vi "UTILITY General Time Header.vi"(6 "precision (6)":i16=6, 7 "Add Elapsed Time (hrs)":bool, 8 "Error In":errorcluster, 9 "Software Elapsed Time":dbl format="%<%H:%M:%S>t", 10 "Elapsed Time":dbl, 11 "Add Software Elapsed Time":bool) -> (0 "Error Out":errorcluster, 3 "Total Array":string[][](array[string]))   [LabVIEW 2020]
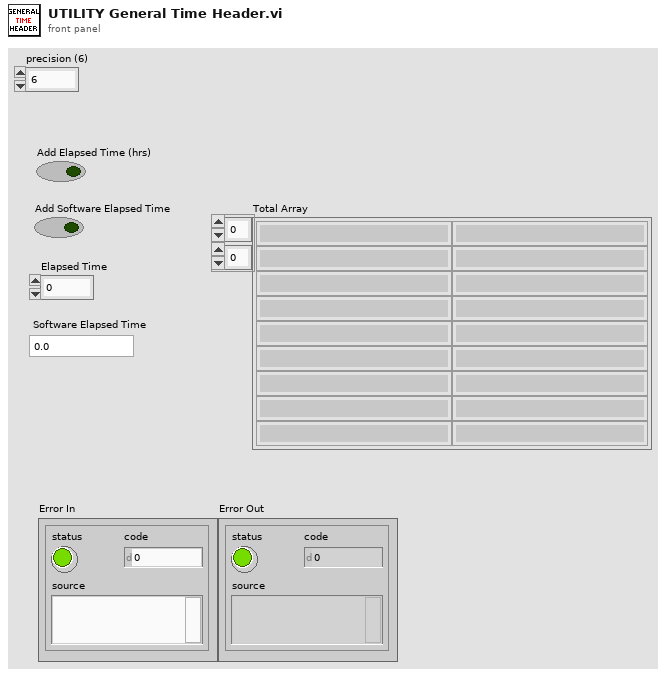
[diagram p1: front panel]
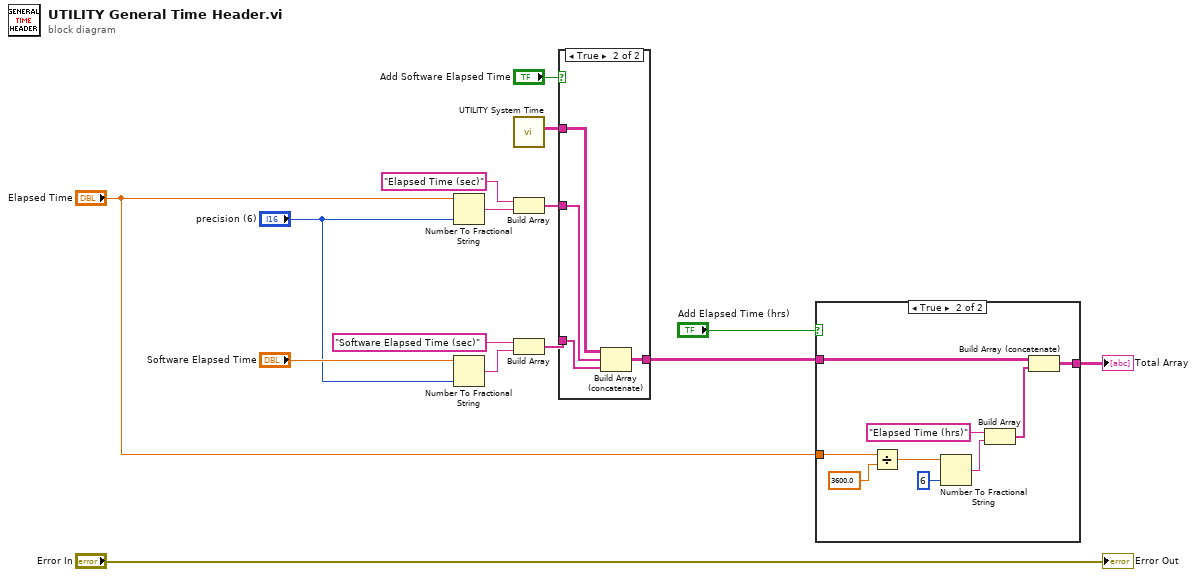
[diagram p0: block diagram]
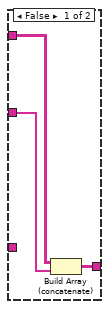
[diagram p3: hidden frame]
diagram:
  n1 = Number To Fractional String(number="Elapsed Time", precision (6)="precision (6)") -> (F-format string=w10:string)  [unwired: 2 in]
  n2 = Number To Fractional String(number="Software Elapsed Time", precision (6)="precision (6)") -> (F-format string=w2:string)  [unwired: 2 in]
  n3 = call "UTILITY System Time.vi"() -> ("Date & Time"=w12:string[][])  [unwired: 10 in, 1 out]
  n4 = Build Array("Elapsed Time (sec)", w10) -> (w11:string[])
  n5 = Build Array("Software Elapsed Time (sec)", w2) -> (w14:string[])
  n6 = case shown="True" "Add Software Elapsed Time" {
    tunnel: w11 -> [w17 w22]
    tunnel: [w16 w21] -> w7
    tunnel: w12 -> [w18 w20]
    tunnel: w14 -> [_ w19]
    frame False {
      n7 = Build Array (concatenate)(w18, w17) -> (w16:string[][])
    }
    frame True {
      n8 = Build Array (concatenate)(w20, w22, w19) -> (w21:string[][])
    }
  }
  n9 = case shown="True" "Add Elapsed Time (hrs)" {
    tunnel: w7 -> [w23 w26]
    tunnel: "Elapsed Time" -> [_ w29]
    tunnel: [w23 w24] -> w4
    frame False {
    }
    frame True {
      n10 = Divide(x=w29, y=3600.0) -> (x/y=w27:dbl)
      n11 = Number To Fractional String(number=w27, precision (6)=i16 6) -> (F-format string=w30:string)  [unwired: 2 in]
      n12 = Build Array("Elapsed Time (hrs)", w30) -> (w25:string[])
      n13 = Build Array (concatenate)(w26, w25) -> (w24:string[][])
    }
  }
  "Total Array" <- w4
  "Error Out" <- "Error In"
